vi "dotNET callback.vi"(4 "queue out":refnum<queue>, 5 "Event Data":cluster{"sender":refnum<k39>, "e":refnum<k39>}, 6 "Control Ref":refnum<k39>, 7 "Event Common Data":T1) -> ()   [LabVIEW 2026]
uses:
  C:/Program Files/dotnet/shared/Microsoft.NETCore.App/8.0.24/System.IO.FileSystem.Watcher.dll
  Program Files/dotnet/shared/Microsoft.NETCore.App/8.0.24/System.IO.FileSystem.Watcher.dll
  C:/Program Files/dotnet/shared/Microsoft.NETCore.App/8.0.24/System.Private.CoreLib.dll
  Program Files/dotnet/shared/Microsoft.NETCore.App/8.0.24/System.Private.CoreLib.dll
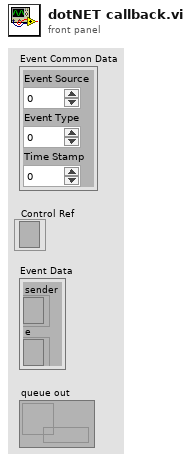
[diagram p1: front panel]
types:
  T1 = cluster{"Event Source":i32, "Event Type":u32, "Time Stamp":u32}
  T2 = cluster{"ChangeType":i32, "FullPath":string, "Name":string}
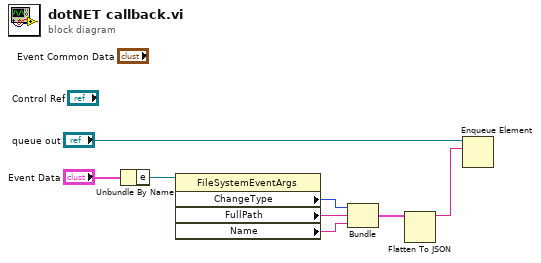
[diagram p0: block diagram]
diagram:
  n1 = Unbundle By Name("Event Data") -> ("e"=w7:refnum<k39>)
  n2 = property class="FileSystemEventArgs"(reference=w7) -> ("ChangeType"=w6:i32, "FullPath"=w5:string, "Name"=w4:string)  [unwired: 1 in, 2 out]
  n3 = Bundle("ChangeType"=w6, "FullPath"=w5, "Name"=w4) -> (w3:T2)  [unwired: 1 in]
  n4 = Flatten To JSON(anything=w3) -> (JSON string=w1:string)  [unwired: 2 in, 1 out]
  n5 = Enqueue Element(queue="queue out", element=w1) -> ()  [unwired: 2 in, 3 out]
